vi "Pian_Virtual_Main.vi"() -> ()   [LabVIEW 2026]
uses:
  <vilib>/Utility/file.llb/Write Delimited Spreadsheet (string).vi
panel:
  in  "Fa#":bool
  in  "Sol#":bool
  in  "La#":bool
  in  "Re#":bool
  in  "Do#":bool
  in  "Salveaza Melodia":bool
  in  "stop":bool
  out "Unda Sonora":dynamicdata(graph)
  in  "Activare Tremolo":bool
  in  "Activare Ecou":bool
  in  "Volum":dbl(knob) scale=0.0..10.0
  in  "Do_sus":bool
  in  "Si":bool
  in  "La":bool
  in  "Sol":bool
  in  "Fa":bool
  in  "Mi":bool
  in  "Re":bool
  in  "Do":bool
  # "Panou de control"
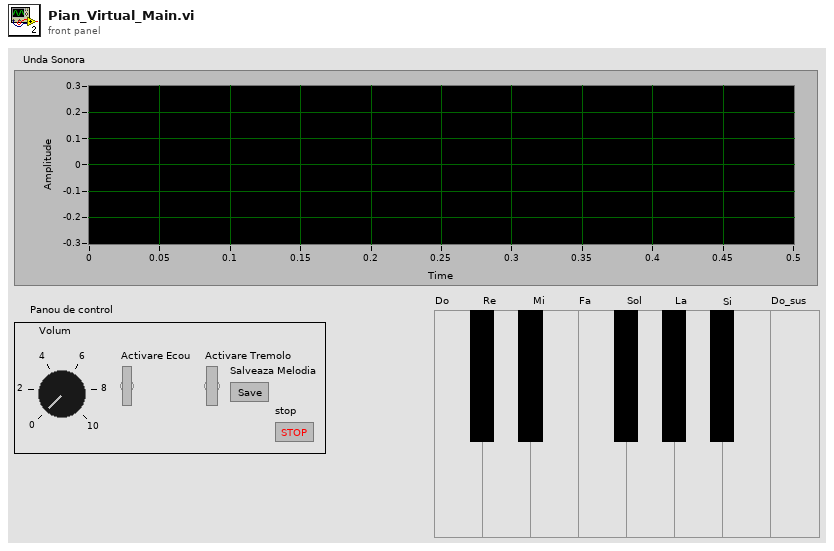
[diagram p1: front panel]
types:
  T1 = enum16{"La#", "Sol#", "Fa#", "Re#", "Do#", "Do_sus", "Si", "La", "Sol", "Fa", "Mi", "Re", "Do"}
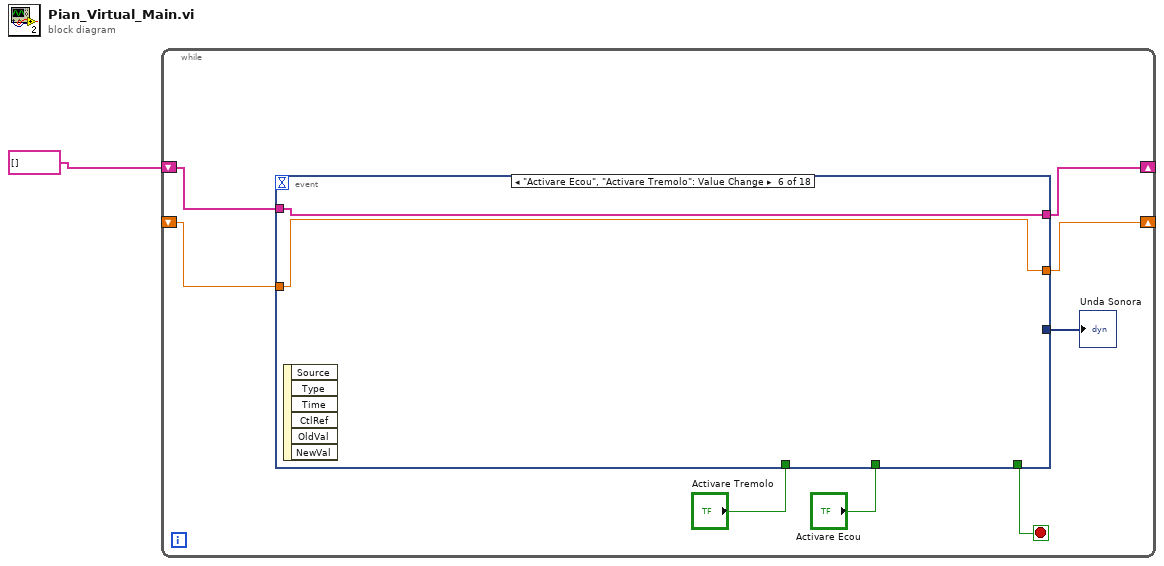
[diagram p0: block diagram]
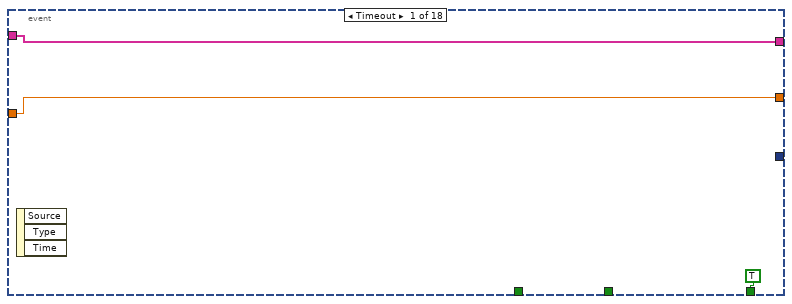
[diagram p2: hidden frame]
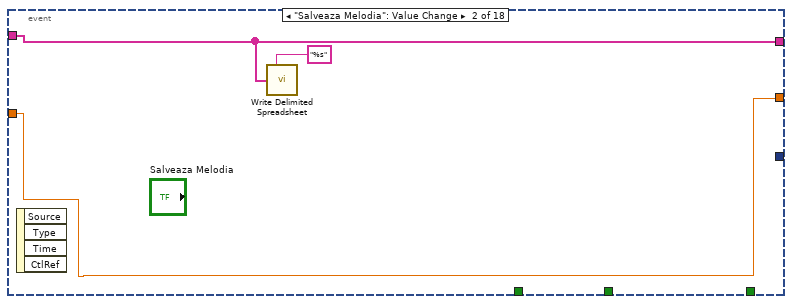
[diagram p3: hidden frame]
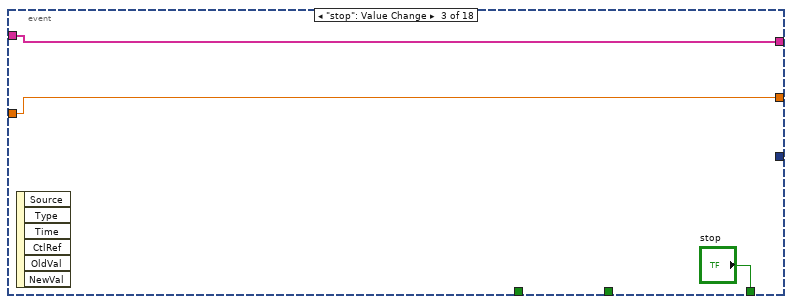
[diagram p4: hidden frame]
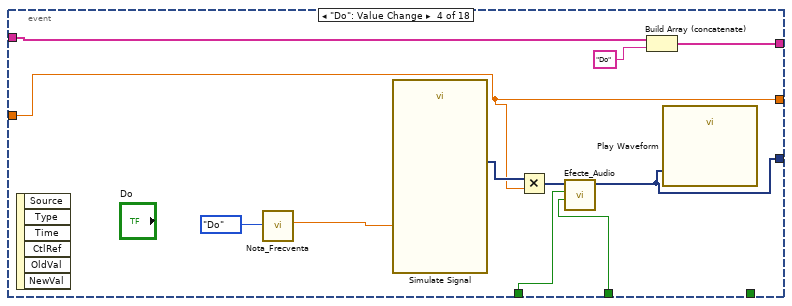
[diagram p5: hidden frame]
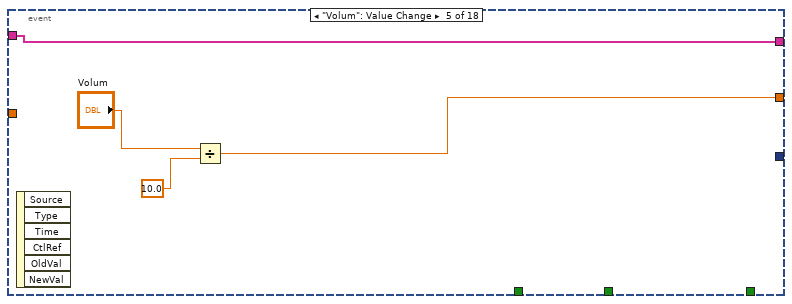
[diagram p6: hidden frame]
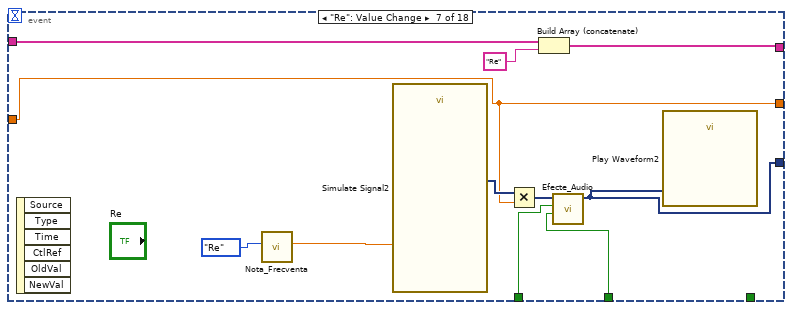
[diagram p7: hidden frame]
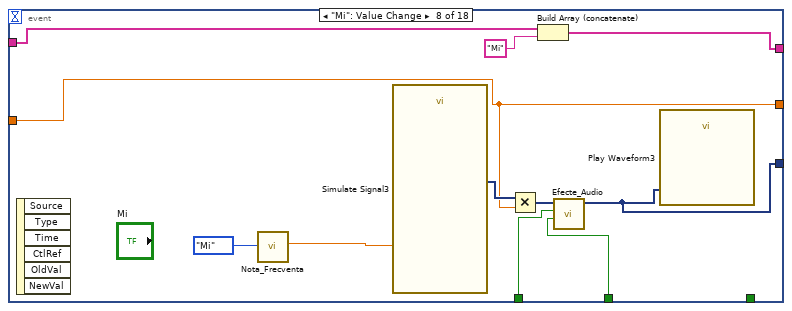
[diagram p8: hidden frame]
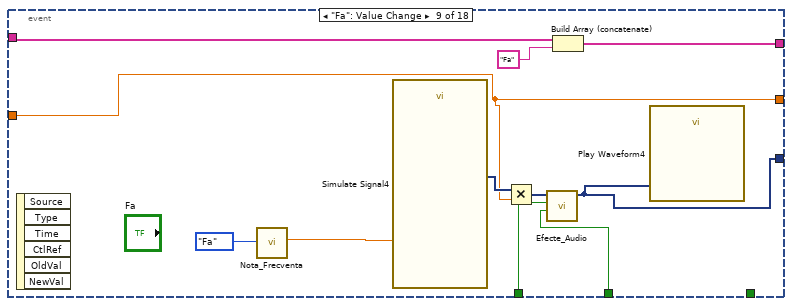
[diagram p9: hidden frame]
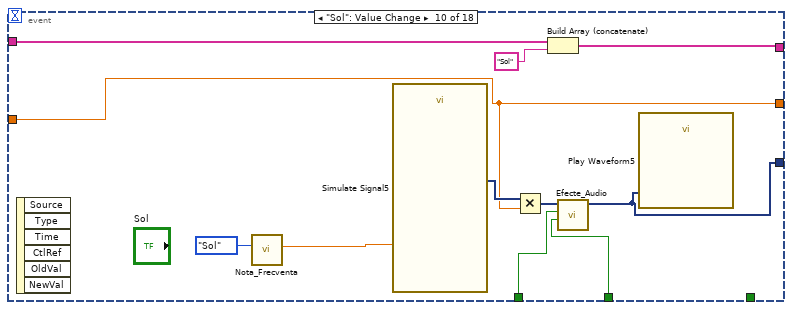
[diagram p10: hidden frame]
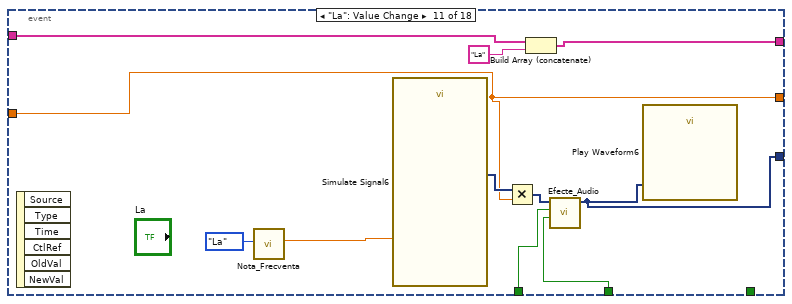
[diagram p11: hidden frame]
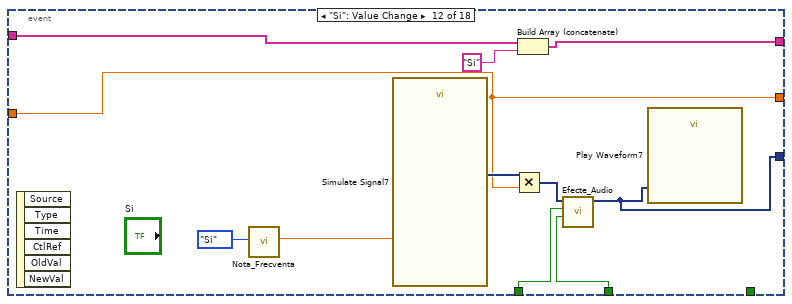
[diagram p12: hidden frame]
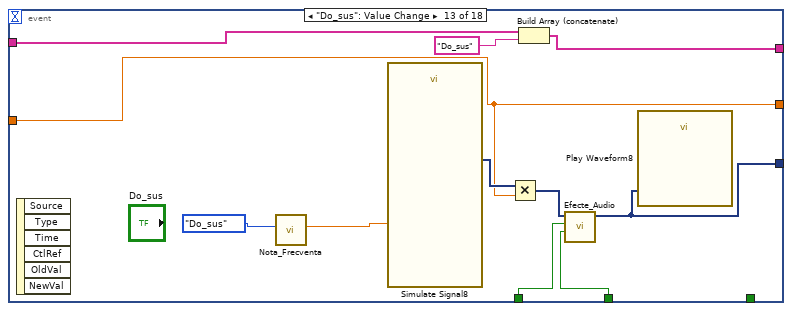
[diagram p13: hidden frame]
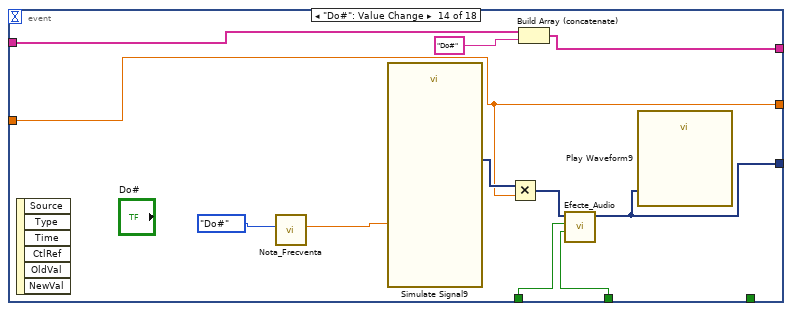
[diagram p14: hidden frame]
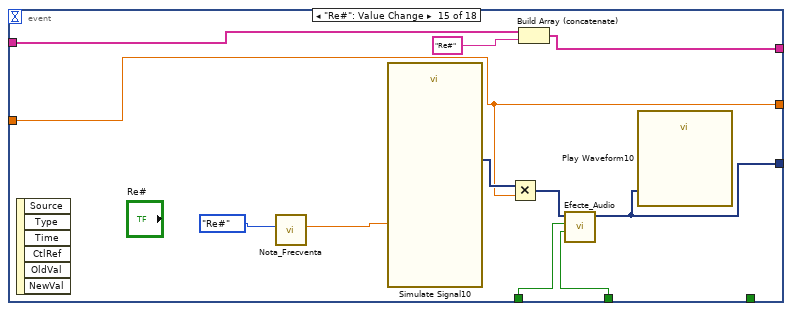
[diagram p15: hidden frame]
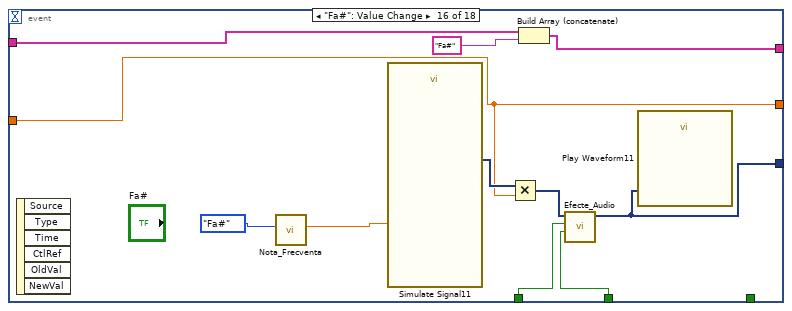
[diagram p16: hidden frame]
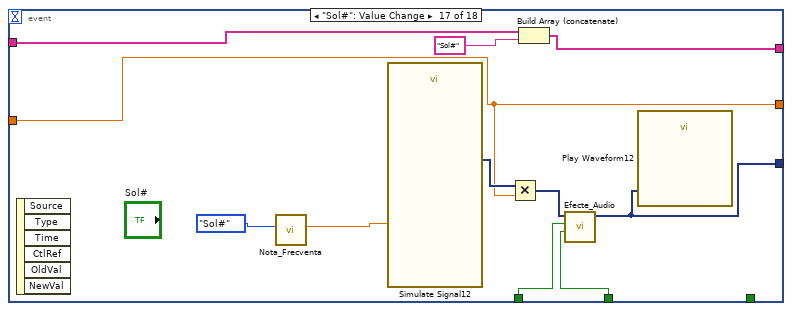
[diagram p17: hidden frame]
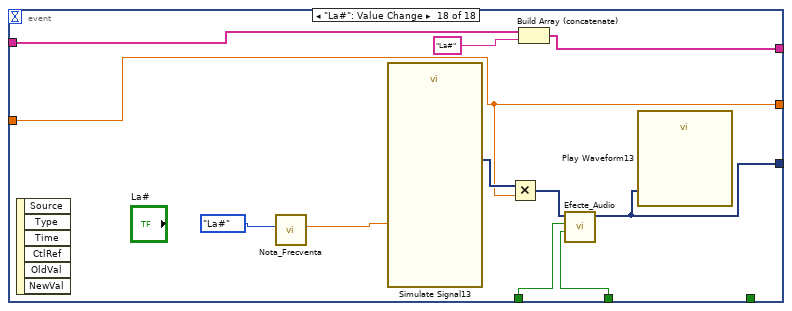
[diagram p18: hidden frame]
diagram:
  n1 = while {
    shift-right: [w6] -> _
    shift-left: _ -> [w7]
    shift-right: [w2] -> _
    shift-left: string[] [] -> [w3]
    stop <- w9 stop-if-true
    n2 = event shown="[5] \"Activare Ecou\", \"Activare Tremolo\": Value Change" {
      selector: _ -> [_ _ _ _ _ _ _ _ _ _ _ _ _ _ _ _ _ _]
      dyn-events: _ -> [_ _ _ _ _ _ _ _ _ _ _ _ _ _ _ _ _ _]
      timeout: _ -> [_ _ _ _ _ _ _ _ _ _ _ _ _ _ _ _ _ _]
      tunnel: [TRUE ("stop") _ "stop" _ _ _ _ _ _ _ _ _ _ _ _ _ _ _] -> w9
      tunnel: [_ _ _ w23 _ _ w40 w51 w62 w73 w84 w95 w107 w118 w129 w140 w151 w162] -> w8
      tunnel: [w11 w15 w17 w27 w31 w34 w44 w55 w66 w77 w88 w99 w109 w120 w131 w142 w153 w164] -> w6
      tunnel: w7 -> [w11 w15 w17 w27 _ w34 w44 w55 w66 w77 w88 w99 w109 w120 w131 w142 w153 w164]
      tunnel: "Activare Tremolo" -> [_ _ _ w25 _ _ w42 w53 w64 w75 w86 w97 w106 w117 w128 w139 w150 w161]
      tunnel: "Activare Ecou" -> [_ _ _ w24 _ _ w41 w52 w63 w74 w85 w96 w105 w116 w127 w138 w149 w160]
      tunnel: w3 -> [w10 w14 w16 w22 w30 w35 w37 w49 w60 w70 w82 w93 w103 w114 w125 w136 w147 w158]
      tunnel: [w10 w14 w16 w21 w30 w35 w38 w48 w59 w71 w81 w92 w102 w113 w124 w135 w146 w157] -> w2
      event Timeout {
        n3 = event-data() -> ()  [unwired: 1 in, 3 out]
      }
      event "Salveaza Melodia": Value Change {
        n4 = event-data() -> ()  [unwired: 1 in, 4 out]
        n5 = call-poly <vilib>:"Write Delimited Spreadsheet.vi"("format (%s)"="%s", "1D data"=w14) -> ()  [unwired: 12 in, 2 out]
      }
      event "stop": Value Change {
        n6 = event-data() -> ()  [unwired: 1 in, 6 out]
      }
      event "Do": Value Change {
        n7 = event-data() -> ()  [unwired: 1 in, 6 out]
        n8 = call "Nota_Frecventa.vi"("Nota Muzicala"=T1."Do") -> ("Frecventa (Hz)"=w29:dbl)  [unwired: 10 in]
        n9 = call "Simulate Signal"("Frequency"=w29) -> ("Sine"=w28:dynamicdata)  [unwired: 13 in, 1 out]
        n10 = Multiply(x=w28, y=w27) -> (x*y=w26:dynamicdata)
        n11 = call "Efecte_Audio.vi"("Activare Ecou"=w24, "Activare Tremolo"=w25, "Semnal Intrare"=w26) -> ("Semnal Iesire"=w23:dynamicdata)  [unwired: 8 in]
        n12 = Build Array (concatenate)(w22, "Do") -> (w21:string[])
        n13 = call "Play Waveform"("Data"=w23) -> ()  [unwired: 18 in, 1 out]
      }
      event "Volum": Value Change {
        n14 = event-data() -> ()  [unwired: 1 in, 6 out]
        n15 = Divide(x="Volum", y=10.0) -> (x/y=w31:dbl)
      }
      event "Activare Ecou", "Activare Tremolo": Value Change {
        n16 = event-data() -> ()  [unwired: 1 in, 6 out]
      }
      event "Re": Value Change {
        n17 = event-data() -> ()  [unwired: 1 in, 6 out]
        n18 = call "Nota_Frecventa.vi"("Nota Muzicala"=T1."Re") -> ("Frecventa (Hz)"=w46:dbl)  [unwired: 10 in]
        n19 = call "Simulate Signal2"("Frequency"=w46) -> ("Sine"=w45:dynamicdata)  [unwired: 13 in, 1 out]
        n20 = Multiply(x=w45, y=w44) -> (x*y=w43:dynamicdata)
        n21 = Build Array (concatenate)(w37, "Re") -> (w38:string[])
        n22 = call "Efecte_Audio.vi"("Activare Ecou"=w41, "Activare Tremolo"=w42, "Semnal Intrare"=w43) -> ("Semnal Iesire"=w40:dynamicdata)  [unwired: 8 in]
        n23 = call "Play Waveform2"("Data"=w40) -> ()  [unwired: 18 in, 1 out]
      }
      event "Mi": Value Change {
        n24 = event-data() -> ()  [unwired: 1 in, 6 out]
        n25 = call "Nota_Frecventa.vi"("Nota Muzicala"=T1."Mi") -> ("Frecventa (Hz)"=w57:dbl)  [unwired: 10 in]
        n26 = call "Simulate Signal3"("Frequency"=w57) -> ("Sine"=w56:dynamicdata)  [unwired: 13 in, 1 out]
        n27 = Multiply(x=w56, y=w55) -> (x*y=w54:dynamicdata)
        n28 = Build Array (concatenate)(w49, "Mi") -> (w48:string[])
        n29 = call "Efecte_Audio.vi"("Activare Ecou"=w52, "Activare Tremolo"=w53, "Semnal Intrare"=w54) -> ("Semnal Iesire"=w51:dynamicdata)  [unwired: 8 in]
        n30 = call "Play Waveform3"("Data"=w51) -> ()  [unwired: 18 in, 1 out]
      }
      event "Fa": Value Change {
        n31 = event-data() -> ()  [unwired: 1 in, 6 out]
        n32 = call "Nota_Frecventa.vi"("Nota Muzicala"=T1."Fa") -> ("Frecventa (Hz)"=w68:dbl)  [unwired: 10 in]
        n33 = call "Simulate Signal4"("Frequency"=w68) -> ("Sine"=w67:dynamicdata)  [unwired: 13 in, 1 out]
        n34 = Multiply(x=w67, y=w66) -> (x*y=w65:dynamicdata)
        n35 = call "Efecte_Audio.vi"("Activare Ecou"=w63, "Activare Tremolo"=w64, "Semnal Intrare"=w65) -> ("Semnal Iesire"=w62:dynamicdata)  [unwired: 8 in]
        n36 = Build Array (concatenate)(w60, "Fa") -> (w59:string[])
        n37 = call "Play Waveform4"("Data"=w62) -> ()  [unwired: 18 in, 1 out]
      }
      event "Sol": Value Change {
        n38 = event-data() -> ()  [unwired: 1 in, 6 out]
        n39 = call "Nota_Frecventa.vi"("Nota Muzicala"=T1."Sol") -> ("Frecventa (Hz)"=w79:dbl)  [unwired: 10 in]
        n40 = call "Simulate Signal5"("Frequency"=w79) -> ("Sine"=w78:dynamicdata)  [unwired: 13 in, 1 out]
        n41 = Multiply(x=w78, y=w77) -> (x*y=w76:dynamicdata)
        n42 = Build Array (concatenate)(w70, "Sol") -> (w71:string[])
        n43 = call "Efecte_Audio.vi"("Activare Ecou"=w74, "Activare Tremolo"=w75, "Semnal Intrare"=w76) -> ("Semnal Iesire"=w73:dynamicdata)  [unwired: 8 in]
        n44 = call "Play Waveform5"("Data"=w73) -> ()  [unwired: 18 in, 1 out]
      }
      event "La": Value Change {
        n45 = event-data() -> ()  [unwired: 1 in, 6 out]
        n46 = call "Nota_Frecventa.vi"("Nota Muzicala"=T1."La") -> ("Frecventa (Hz)"=w90:dbl)  [unwired: 10 in]
        n47 = call "Simulate Signal6"("Frequency"=w90) -> ("Sine"=w89:dynamicdata)  [unwired: 13 in, 1 out]
        n48 = Multiply(x=w89, y=w88) -> (x*y=w87:dynamicdata)
        n49 = Build Array (concatenate)(w82, "La") -> (w81:string[])
        n50 = call "Efecte_Audio.vi"("Activare Ecou"=w85, "Activare Tremolo"=w86, "Semnal Intrare"=w87) -> ("Semnal Iesire"=w84:dynamicdata)  [unwired: 8 in]
        n51 = call "Play Waveform6"("Data"=w84) -> ()  [unwired: 18 in, 1 out]
      }
      event "Si": Value Change {
        n52 = event-data() -> ()  [unwired: 1 in, 6 out]
        n53 = call "Nota_Frecventa.vi"("Nota Muzicala"=T1."Si") -> ("Frecventa (Hz)"=w101:dbl)  [unwired: 10 in]
        n54 = call "Simulate Signal7"("Frequency"=w101) -> ("Sine"=w100:dynamicdata)  [unwired: 13 in, 1 out]
        n55 = Multiply(x=w100, y=w99) -> (x*y=w98:dynamicdata)
        n56 = Build Array (concatenate)(w93, "Si") -> (w92:string[])
        n57 = call "Efecte_Audio.vi"("Activare Ecou"=w96, "Activare Tremolo"=w97, "Semnal Intrare"=w98) -> ("Semnal Iesire"=w95:dynamicdata)  [unwired: 8 in]
        n58 = call "Play Waveform7"("Data"=w95) -> ()  [unwired: 18 in, 1 out]
      }
      event "Do_sus": Value Change {
        n59 = event-data() -> ()  [unwired: 1 in, 6 out]
        n60 = call "Nota_Frecventa.vi"("Nota Muzicala"=T1."Do_sus") -> ("Frecventa (Hz)"=w111:dbl)  [unwired: 10 in]
        n61 = call "Simulate Signal8"("Frequency"=w111) -> ("Sine"=w110:dynamicdata)  [unwired: 13 in, 1 out]
        n62 = Multiply(x=w110, y=w109) -> (x*y=w108:dynamicdata)
        n63 = Build Array (concatenate)(w103, "Do_sus") -> (w102:string[])
        n64 = call "Efecte_Audio.vi"("Activare Ecou"=w105, "Activare Tremolo"=w106, "Semnal Intrare"=w108) -> ("Semnal Iesire"=w107:dynamicdata)  [unwired: 8 in]
        n65 = call "Play Waveform8"("Data"=w107) -> ()  [unwired: 18 in, 1 out]
      }
      event "Do#": Value Change {
        n66 = event-data() -> ()  [unwired: 1 in, 6 out]
        n67 = call "Nota_Frecventa.vi"("Nota Muzicala"=T1."Do#") -> ("Frecventa (Hz)"=w122:dbl)  [unwired: 10 in]
        n68 = call "Simulate Signal9"("Frequency"=w122) -> ("Sine"=w121:dynamicdata)  [unwired: 13 in, 1 out]
        n69 = Multiply(x=w121, y=w120) -> (x*y=w119:dynamicdata)
        n70 = Build Array (concatenate)(w114, "Do#") -> (w113:string[])
        n71 = call "Efecte_Audio.vi"("Activare Ecou"=w116, "Activare Tremolo"=w117, "Semnal Intrare"=w119) -> ("Semnal Iesire"=w118:dynamicdata)  [unwired: 8 in]
        n72 = call "Play Waveform9"("Data"=w118) -> ()  [unwired: 18 in, 1 out]
      }
      event "Re#": Value Change {
        n73 = event-data() -> ()  [unwired: 1 in, 6 out]
        n74 = call "Nota_Frecventa.vi"("Nota Muzicala"=T1."Re#") -> ("Frecventa (Hz)"=w133:dbl)  [unwired: 10 in]
        n75 = call "Simulate Signal10"("Frequency"=w133) -> ("Sine"=w132:dynamicdata)  [unwired: 13 in, 1 out]
        n76 = Multiply(x=w132, y=w131) -> (x*y=w130:dynamicdata)
        n77 = Build Array (concatenate)(w125, "Re#") -> (w124:string[])
        n78 = call "Efecte_Audio.vi"("Activare Ecou"=w127, "Activare Tremolo"=w128, "Semnal Intrare"=w130) -> ("Semnal Iesire"=w129:dynamicdata)  [unwired: 8 in]
        n79 = call "Play Waveform10"("Data"=w129) -> ()  [unwired: 18 in, 1 out]
      }
      event "Fa#": Value Change {
        n80 = event-data() -> ()  [unwired: 1 in, 6 out]
        n81 = call "Nota_Frecventa.vi"("Nota Muzicala"=T1."Fa#") -> ("Frecventa (Hz)"=w144:dbl)  [unwired: 10 in]
        n82 = call "Simulate Signal11"("Frequency"=w144) -> ("Sine"=w143:dynamicdata)  [unwired: 13 in, 1 out]
        n83 = Multiply(x=w143, y=w142) -> (x*y=w141:dynamicdata)
        n84 = Build Array (concatenate)(w136, "Fa#") -> (w135:string[])
        n85 = call "Efecte_Audio.vi"("Activare Ecou"=w138, "Activare Tremolo"=w139, "Semnal Intrare"=w141) -> ("Semnal Iesire"=w140:dynamicdata)  [unwired: 8 in]
        n86 = call "Play Waveform11"("Data"=w140) -> ()  [unwired: 18 in, 1 out]
      }
      event "Sol#": Value Change {
        n87 = event-data() -> ()  [unwired: 1 in, 6 out]
        n88 = call "Nota_Frecventa.vi"("Nota Muzicala"=T1."Sol#") -> ("Frecventa (Hz)"=w155:dbl)  [unwired: 10 in]
        n89 = call "Simulate Signal12"("Frequency"=w155) -> ("Sine"=w154:dynamicdata)  [unwired: 13 in, 1 out]
        n90 = Multiply(x=w154, y=w153) -> (x*y=w152:dynamicdata)
        n91 = Build Array (concatenate)(w147, "Sol#") -> (w146:string[])
        n92 = call "Efecte_Audio.vi"("Activare Ecou"=w149, "Activare Tremolo"=w150, "Semnal Intrare"=w152) -> ("Semnal Iesire"=w151:dynamicdata)  [unwired: 8 in]
        n93 = call "Play Waveform12"("Data"=w151) -> ()  [unwired: 18 in, 1 out]
      }
      event "La#": Value Change {
        n94 = event-data() -> ()  [unwired: 1 in, 6 out]
        n95 = call "Nota_Frecventa.vi"("Nota Muzicala"=T1."La#") -> ("Frecventa (Hz)"=w166:dbl)  [unwired: 10 in]
        n96 = call "Simulate Signal13"("Frequency"=w166) -> ("Sine"=w165:dynamicdata)  [unwired: 13 in, 1 out]
        n97 = Multiply(x=w165, y=w164) -> (x*y=w163:dynamicdata)
        n98 = Build Array (concatenate)(w158, "La#") -> (w157:string[])
        n99 = call "Efecte_Audio.vi"("Activare Ecou"=w160, "Activare Tremolo"=w161, "Semnal Intrare"=w163) -> ("Semnal Iesire"=w162:dynamicdata)  [unwired: 8 in]
        n100 = call "Play Waveform13"("Data"=w162) -> ()  [unwired: 18 in, 1 out]
      }
    }
    "Unda Sonora" <- w8
  }
